vi "save log file auto.vi"(0 "log array":string[][](array[string])) -> ()   [LabVIEW 2019]
uses:
  <vilib>/Utility/file.llb/Write To Spreadsheet File (string).vi
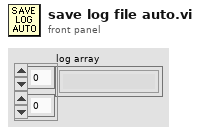
[diagram p1: front panel]
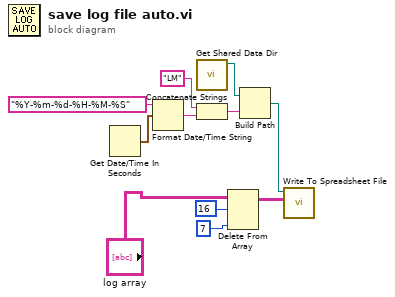
[diagram p0: block diagram]
diagram:
  n1 = Get Date/Time In Seconds() -> (seconds since 1Jan1904=w9:timestamp)
  n2 = Format Date/Time String(time format string (%c)="%Y-%m-%d-%H-%M-%S", seconds (now)=w9) -> (date/time string=w11:string)  [unwired: 1 in]
  n3 = call "Get Shared Data Dir.vi"() -> ("Data Directory Path"=w6:path)  [unwired: 2 in, 1 out]
  n4 = Concatenate Strings("LM" ("string"), w11) -> (w7:string)
  n5 = Delete From Array(array="log array", length=16 ("disabled index (col)"), index (col)=7 ("disabled index (col)")) -> (array with subset deleted=w2:string[][])  [unwired: 1 in, 1 out]
  n6 = Build Path(base path=w6, name or relative path=w7) -> (appended path=w8:path)
  n7 = call-poly <vilib>:"Write To Spreadsheet File.vi"("2D data"=w2, "file path (dialog if empty)"=w8) -> ()  [unwired: 6 in, 1 out]
